vi "Find Child of Node By Key.vi"(8 "error in":errorcluster, 9 "Key":string, 10 "Node":T1={"Record Type"="BGNSTR", "Payload"="\u0000b\u0000\b\u0000\u0019\u0000\u000f\u00005\u0000\f\u0000b\u0000\b\u0000\u0019\u0000\u000f\u00005\u0000\f", "Parent Index"=0, "First Child Index"=6, "Next Sibling Index"=13}, 11 "Fast Tree in":refnum<class "Fast Tree.lvclass">) -> (0 "error out":errorcluster, 1 "Found?":bool, 2 "Child":T1, 3 "Fast Tree out":refnum<class "Fast Tree.lvclass">)   [LabVIEW 2019, in "Fast Tree.lvclass"]
uses:
  Fast Tree.lvclass
  Fast Tree.lvclass/Fast Tree.ctl
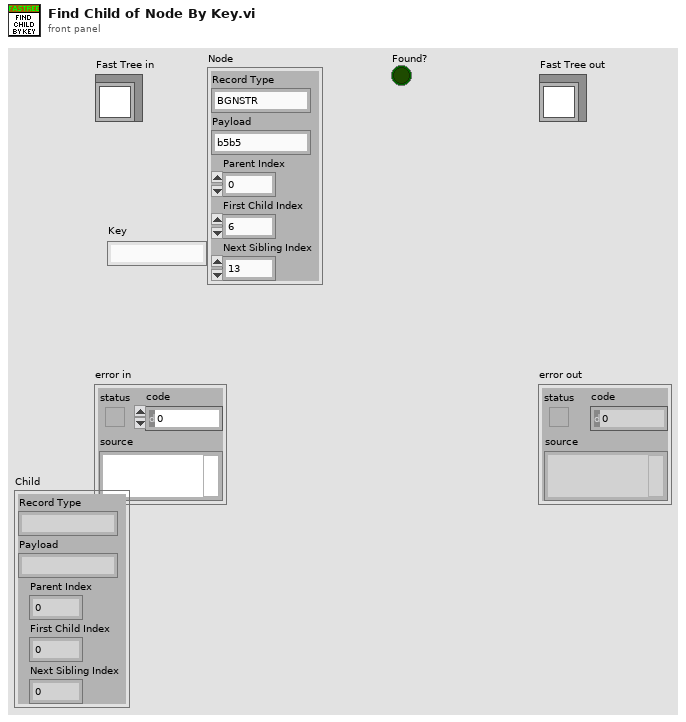
[diagram p1: front panel]
types:
  T1 = cluster{"Record Type":string, "Payload":string, "Parent Index":i32, "First Child Index":i32, "Next Sibling Index":i32}
  T2 = cluster{"Record Type":string, "Payload":string, "Parent Index":i32, "First Child Index":i32, "Next Sibling Index":i32}[]
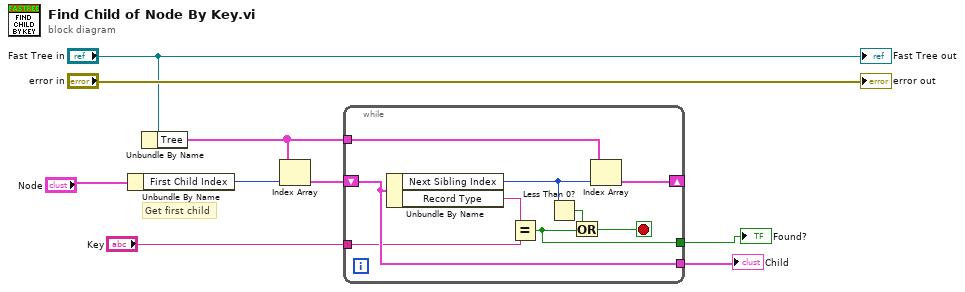
[diagram p0: block diagram]
diagram:
  # "Get first child"
  n1 = Unbundle By Name("Node") -> ("First Child Index"=w6:i32)
  n2 = Unbundle By Name("Fast Tree in") -> ("Tree"=w7:T2)
  n3 = Index Array(array=w7, index=w6) -> (element=w8:T1)
  n4 = while {
    tunnel: [w18] -> w1
    tunnel: w7 -> [w17]
    shift-right: [w16] -> _
    shift-left: w8 -> [w18]
    tunnel: "Key" -> [w13]
    tunnel: [w10] -> w2
    stop <- w11 stop-if-true
    n5 = Unbundle By Name(w18) -> ("Next Sibling Index"=w15:i32, "Record Type"=w14:string)
    n6 = Equal?(x=w14, y=w13) -> (x = y?=w10:bool)
    n7 = Less Than 0?(x=w15) -> (x < 0?=w12:bool)
    n8 = Or(x=w12, y=w10) -> (x .or. y?=w11:bool)
    n9 = Index Array(array=w17, index=w15) -> (element=w16:T1)
  }
  "Child" <- w1
  "Found?" <- w2
  "error out" <- "error in"
  "Fast Tree out" <- "Fast Tree in"
